vi "State Elapsed Time.vi"(7 "State Machine":enum16{"Transfer Sample", "Push Sample"}(ring), 8 "error in (no error)":errorcluster, 10 "Reset (F)":bool caption="Reset", 11 "cRIO-CO2 in":refnum<class "cRIO-CO2.lvclass">) -> (0 "error out":errorcluster, 1 "State Timeout?":bool caption="Time has Elapsed", 2 "Elapsed Time (s)":dbl, 3 "cRIO-CO2 out":refnum<class "cRIO-CO2.lvclass">)   [LabVIEW 2015, in "cRIO-Carbondioxide.lvlib" / "cRIO-CO2.lvlib" / "cRIO-CO2.lvclass"]
uses:
  cRIO-CO2.lvclass
  cRIO-CO2.lvclass/cRIO-CO2.ctl
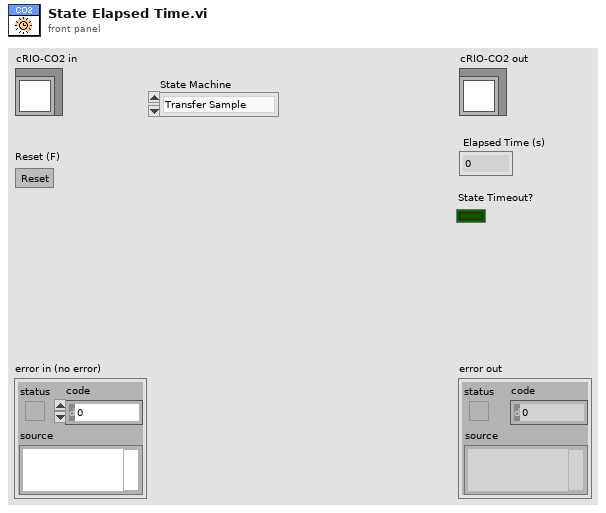
[diagram p1: front panel]
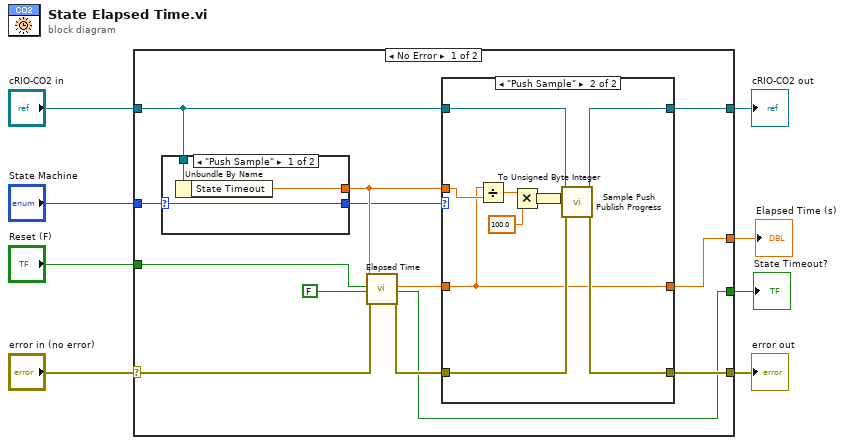
[diagram p0: block diagram]
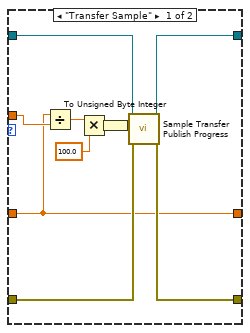
[diagram p2: hidden frame]
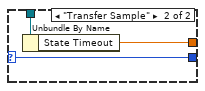
[diagram p3: hidden frame]
diagram:
  n1 = case shown="No Error" "error in (no error)" {
    selector: "error in (no error)" -> [w21 w49]
    tunnel: [w14 w49] -> w7
    tunnel: [w16 w48] -> w5
    tunnel: "cRIO-CO2 in" -> [w17 w48]
    tunnel: [w10 _] -> w4
    tunnel: [w9 _] -> w3
    tunnel: "Reset (F)" -> [w18 _]
    tunnel: "State Machine" -> [w19 _]
    frame No Error {
      n2 = case shown="\"Push Sample\"" w19 {
        selector: w19 -> [w42 w45]
        tunnel: [w44 w47] -> w13
        tunnel: w17 -> [w43 w46]
        tunnel: [w42 w45] -> w11
        frame "Push Sample" {
          n3 = Unbundle By Name(w43) -> ("State Timeout"=w44:dbl)
        }
        frame "Transfer Sample" {
          n4 = Unbundle By Name(w46) -> ("State Timeout"=w47:dbl)
        }
      }
      n5 = call "Elapsed Time"("Time Target (s)"=w13, "Reset"=w18, "Auto Reset"=FALSE, "error in (no error)"=w21) -> ("Elapsed Time (s)"=w12:dbl, "Time has Elapsed"=w10:bool, "error out"=w15:errorcluster)  [unwired: 8 in, 5 out]
      n6 = case shown="\"Push Sample\"" w11 {
        tunnel: w17 -> [w31 w41]
        tunnel: [w30 w40] -> w16
        tunnel: w15 -> [w29 w39]
        tunnel: [w28 w38] -> w14
        tunnel: w13 -> [w27 w37]
        tunnel: w12 -> [w22 w32]
        tunnel: [w22 w32] -> w9
        frame "Transfer Sample" {
          n7 = Divide(x=w22, y=w27) -> (x/y=w25:dbl)
          n8 = Multiply(x=w25, y=100.0) -> (x*y=w26:dbl)
          n9 = To Unsigned Byte Integer(number=w26) -> (unsigned 8bit integer=w23:u8)
          n10 = call "Sample Transfer Publish Progress.vi"("error in (no error)"=w29, "Progress"=w23, "cRIO-CO2 in"=w31) -> ("error out"=w28:errorcluster, "cRIO-CO2 out"=w30:refnum<class "cRIO-CO2.lvclass">)  [unwired: 7 in]
        }
        frame "Push Sample" {
          n11 = Divide(x=w32, y=w37) -> (x/y=w35:dbl)
          n12 = Multiply(x=w35, y=100.0) -> (x*y=w36:dbl)
          n13 = To Unsigned Byte Integer(number=w36) -> (unsigned 8bit integer=w33:u8)
          n14 = call "Sample Push Publish Progress.vi"("error in (no error)"=w39, "Progress"=w33, "cRIO-CO2 in"=w41) -> ("error out"=w38:errorcluster, "cRIO-CO2 out"=w40:refnum<class "cRIO-CO2.lvclass">)  [unwired: 7 in]
        }
      }
    }
    frame Error {
    }
  }
  "error out" <- w7
  "cRIO-CO2 out" <- w5
  "State Timeout?" <- w4
  "Elapsed Time (s)" <- w3
